vi "Poll_Data_Main_v2.vi"(8 "error in":errorcluster, 11 "Resources in":T2 {"ZI ModHandle"."ModHandle" format="0x%08x"; "ZI ModHandle"."Conn" format="0x%08x"; "ZI Handle"."Handle" format="0x%08x"; "ZI Handle"."Conn" format="0x%08x"}) -> (0 "error out":errorcluster, 1 "ZI Data 3":T1, 2 "ZI Data 0":T1, 3 "Resources out":T2 {"ZI ModHandle"."ModHandle" format="0x%08x"; "ZI ModHandle"."Conn" format="0x%08x"; "ZI Handle"."Handle" format="0x%08x"; "ZI Handle"."Conn" format="0x%08x"})   [LabVIEW 2021]
uses:
  Resources_v2.ctl
  <instrlib>/Zurich Instruments LabOne/Public/ziTypeHandle.ctl
  <instrlib>/Zurich Instruments LabOne/Public/Modules/ziTypeModHandle.ctl
  ZI_Data_v2.ctl
  <instrlib>/Zurich Instruments LabOne/Public/Modules/ziModGetDoubleData.vi
  <instrlib>/Zurich Instruments LabOne/Public/Utility/ziTicksToS_vector.vi
  <instrlib>/Zurich Instruments LabOne/Zurich Instruments LabOne.lvlib
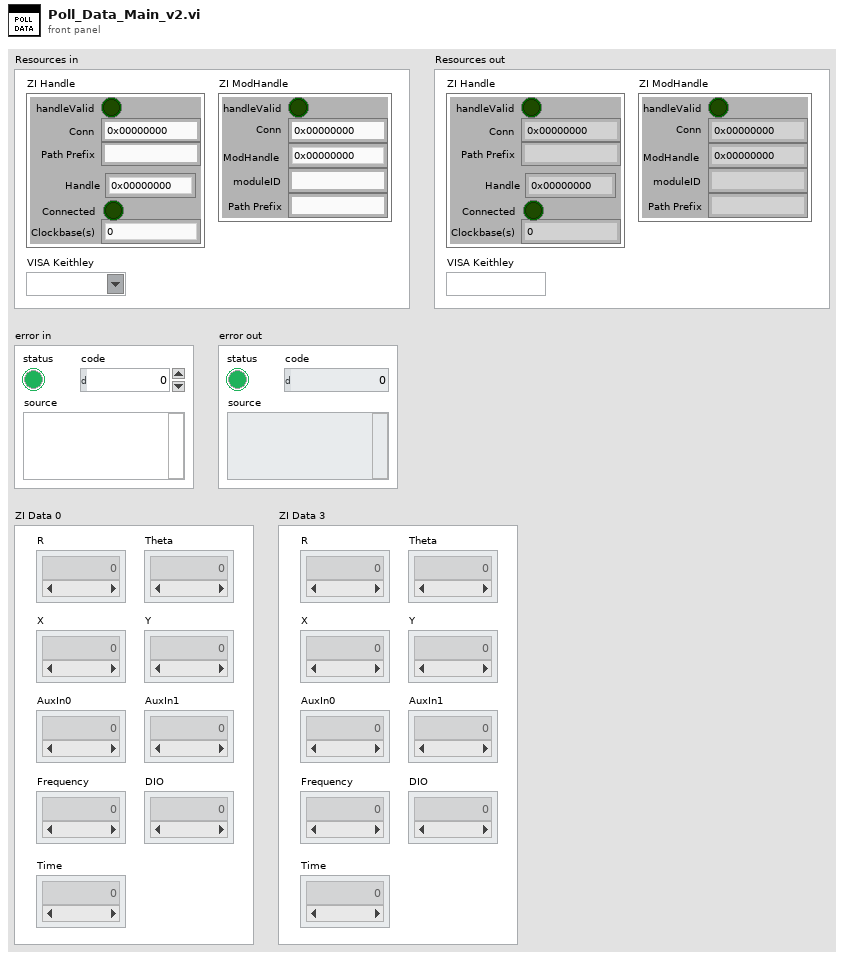
[diagram p1: front panel]
types:
  T1 = typedef "ZI_Data_v2.ctl" = cluster{"R":dbl[], "Theta":dbl[], "X":dbl[], "Y":dbl[], "AuxIn0":dbl[], "AuxIn1":dbl[], "Frequency":dbl[], "DIO":dbl[], "Time":dbl[]}
  T2 = typedef "Resources_v2.ctl" = cluster{"ZI Handle":T3, "ZI ModHandle":T4, "VISA Keithley":refnum<visa-resource-name>}
  T3 = typedef "Zurich Instruments LabOne.lvlib/ziTypeHandle.ctl" = cluster{"handleValid":bool, "Conn":u64, "Path Prefix":string, "Handle":u64, "Clockbase(s)":dbl, "Connected":bool}
  T4 = typedef "Zurich Instruments LabOne.lvlib/ziTypeModHandle.ctl" = cluster{"handleValid":bool, "Conn":u64, "ModHandle":u64, "moduleID":string, "Path Prefix":string}
  T5 = typedef "Zurich Instruments LabOne.lvlib/ziTypeModResults.ctl" = cluster{"PathArray":string[], "ValueType":T6, "NoOfResults":u64, "ziGenericHeader":T7[]}
  T6 = typedef "Zurich Instruments LabOne.lvlib/ziTypePollType.ctl" = enum16{"NONE", "DOUBLE_DATA", "INTEGER_DATA", "DEMOD_SAMPLE", "SCOPE_WAVE_HF2", "AUXIN_SAMPLE", "DIO_SAMPLE", "BYTE_ARRAY", "PWA_WAVE", "9", "10", "11", "12", "13", "14", "15", "TREE_CHANGE_DEPRI", "17", "ERROR", "19", "20", "21", "22", "23", "24", "25", "26", "27", "28", "29", "30", "31", "DOUBLE_DATA_TS", "INTEGER_DATA_TS", "34", "SCOPE_WAVE", "SCOPE_WAVE_EX", "37", "BYTE_ARRAY_TS", "39", "40", "41", "42", "43", "44", "45", "CNT_DATA", "47", "TREE_CHANGE", "49", "50", "51", "52", "53", "54", "55", "56", "57", "58", "59", "60", "61", "62", "63", "SWEEPER_DATA", "SPECTRUM_DATA", "ADVISOR_DATA", "VECTOR_DATA", "IMP_DATA"}
  T7 = typedef "Zurich Instruments LabOne.lvlib/ziTypeModGenericHeader.ctl" = cluster{"HeaderType":enum8{"HEADER_TYPE_NONE", "HEADER_TYPE_SWTRIGGER", "HEADER_TYPE_SWEEPER"}, "SampleFormat":u8, "SystemTime":timestamp, "CreatedTimeStamp":u64, "ChangedTimeStamp":u64, "Flags":u32, "ChunkSizeBytes":u64, "Name":string, "Status":u32, "GroupIndex":u32, "Color":u32, "ActiveRow":u32, "TriggerNumber":u64, "GridRows":u32, "GridCols":u32, "GridMode":u32, "GridOperation":u32, "GridDirection":u32, "GridRepetitions":u32, "GridColDelta":dbl, "GridColOffset":dbl, "GridRowDelta":dbl, "GridRowOffset":dbl, "Bandwidth":dbl, "Center":dbl, "Nenbw":dbl}
  T8 = typedef "Zurich Instruments LabOne.lvlib/ziTypeDoubleDataTS.ctl" = cluster{"Timestamp (ticks)":u64[], "Value":dbl[]}
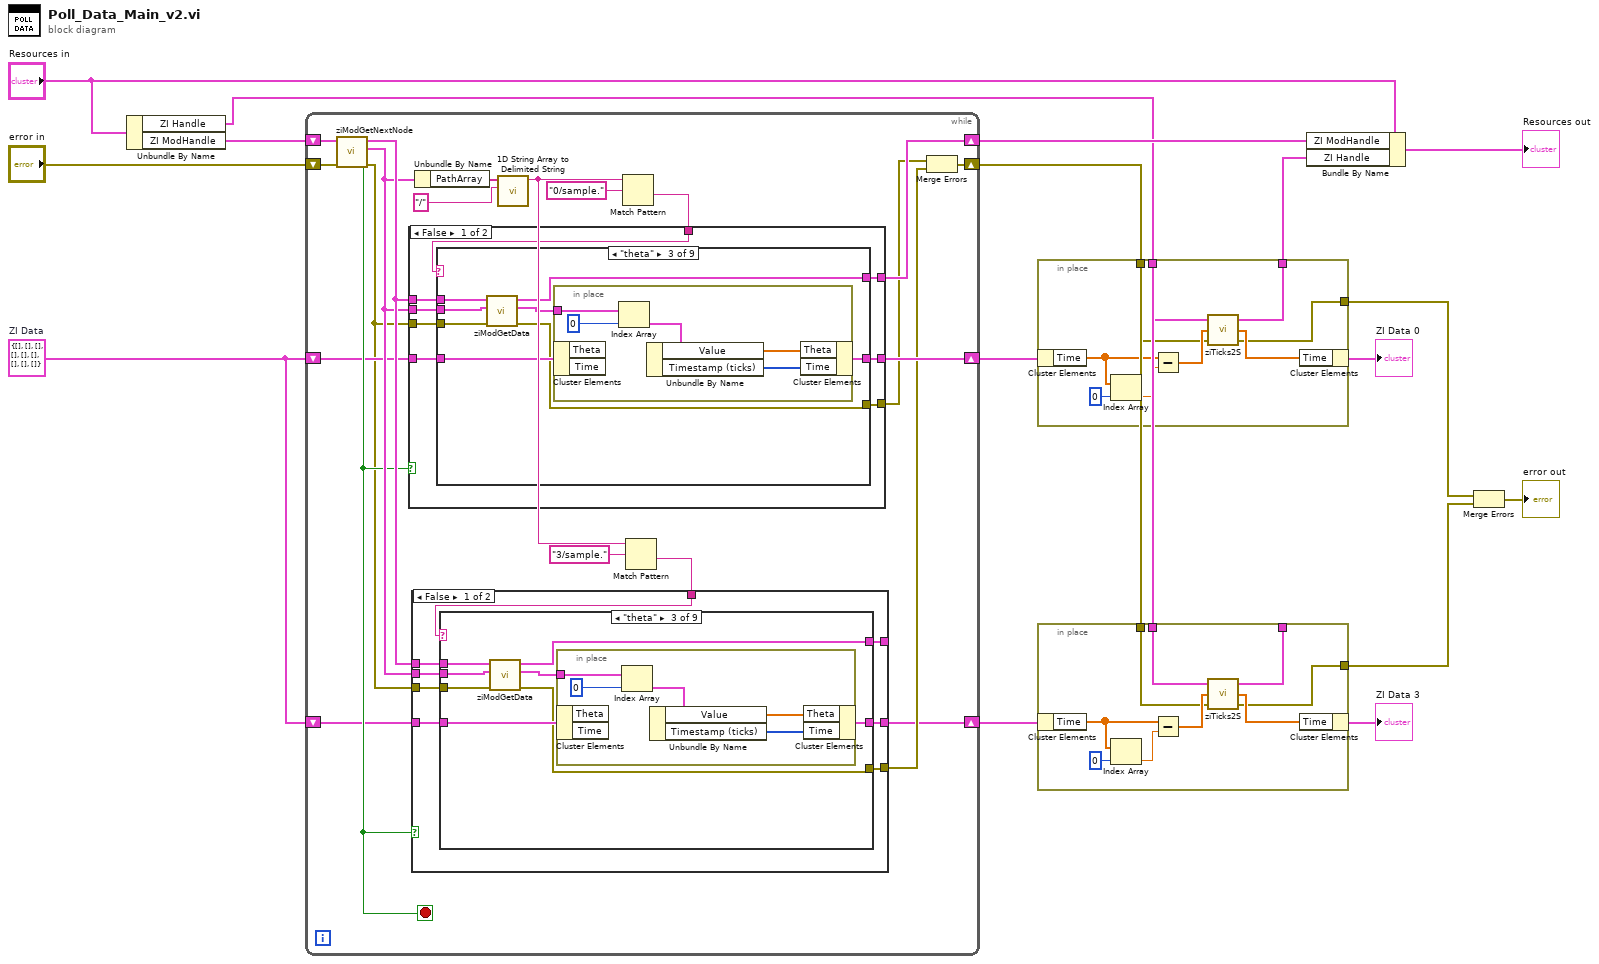
[diagram p0: block diagram]
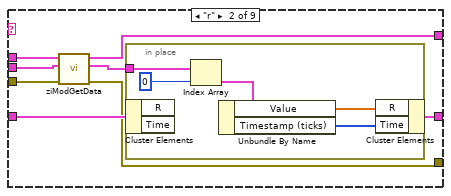
[diagram p3: hidden frame]
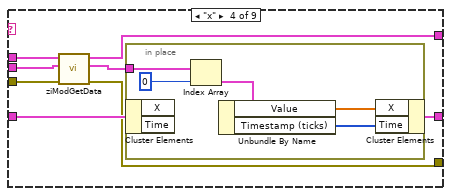
[diagram p4: hidden frame]
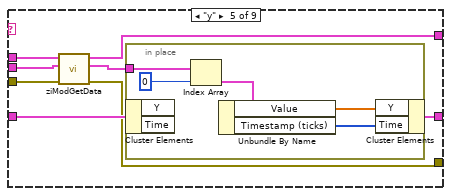
[diagram p5: hidden frame]
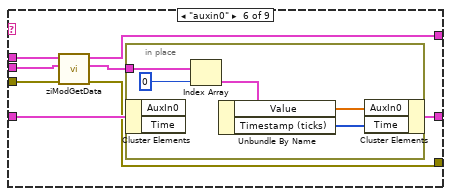
[diagram p6: hidden frame]
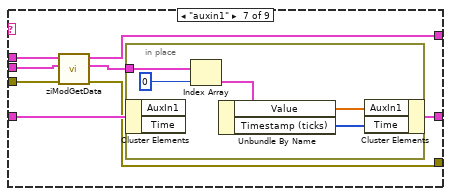
[diagram p7: hidden frame]
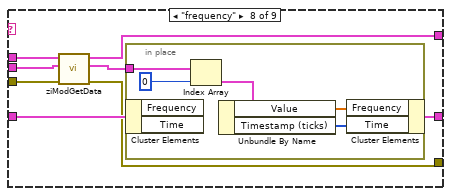
[diagram p8: hidden frame]
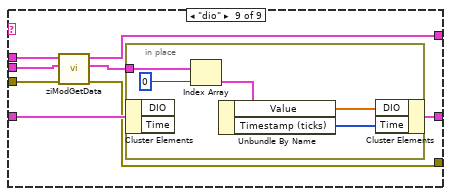
[diagram p9: hidden frame]
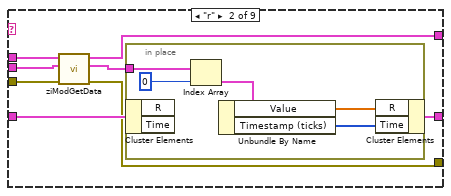
[diagram p12: hidden frame]
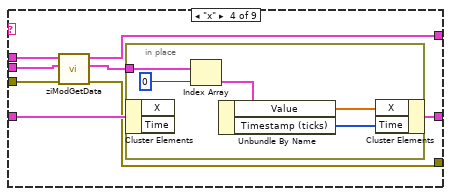
[diagram p13: hidden frame]
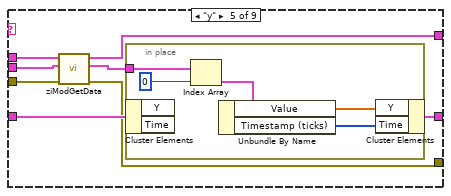
[diagram p14: hidden frame]
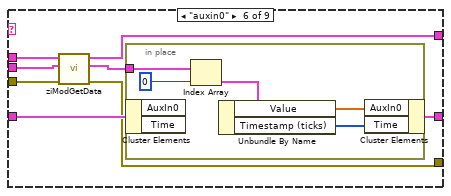
[diagram p15: hidden frame]
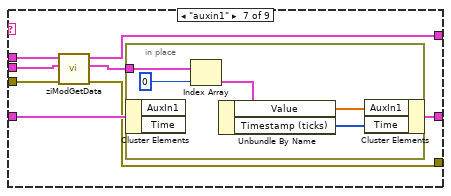
[diagram p16: hidden frame]
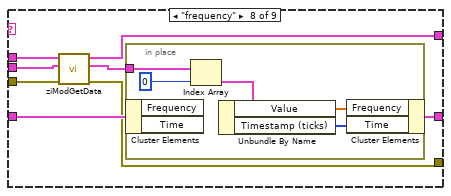
[diagram p17: hidden frame]
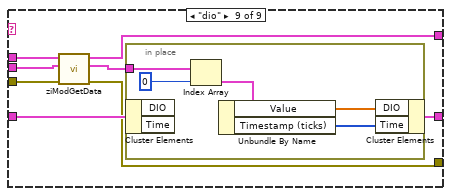
[diagram p18: hidden frame]
diagram:
  w3 = T1 {"R"=[], "Theta"=[], "X"=[], "Y"=[], "AuxIn0"=[], "AuxIn1"=[], "Frequency"=[], "DIO"=[], "Time"=[]}  # ZI Data
  n1 = Unbundle By Name("Resources in") -> ("ZI Handle"=w11:T3, "ZI ModHandle"=w13:T4)
  n2 = while {
    shift-right: [w31] -> w16
    shift-left: w13 -> [w37]
    shift-right: [w19] -> w6
    shift-left: "error in" -> [w36]
    shift-right: [w32] -> w15
    shift-left: w3 -> [w23]
    shift-right: [w17] -> w7
    shift-left: w3 -> [w18]
    stop <- w24 stop-if-true
    n3 = call <instrlib>:"ziModGetNextNode.vi"("Error In"=w36, "ModHandle In"=w37) -> ("Error Out"=w22:errorcluster, "ModResults"=w25:T5, "ModHandle Out"=w26:T4, "NoData"=w24:bool)  [unwired: 6 in]
    n4 = Unbundle By Name(w25) -> ("PathArray"=w33:string[])
    n5 = call <vilib>:"1D String Array to Delimited String.vi"("delimiter"="/", "string array"=w33) -> ("delimited string"=w27:string)  [unwired: 9 in]
    n6 = Match Pattern(string=w27, regular expression="0/sample.") -> (after substring=w30:string)  [unwired: 1 in, 3 out]
    n7 = case shown="False" w24 {
      tunnel: w30 -> [w163 _]
      tunnel: w22 -> [w161 w272]
      tunnel: w26 -> [w162 w271]
      tunnel: w25 -> [w160 _]
      tunnel: w23 -> [w159 w273]
      tunnel: [w158 w273] -> w32
      tunnel: [w157 w271] -> w31
      tunnel: [w156 w272] -> w21
      frame False {
        n8 = case shown="\"theta\"" w163 {
          tunnel: w162 -> [w166 w174 w187 w200 w213 w226 w239 w252 w265]
          tunnel: w161 -> [w164 w173 w186 w199 w212 w225 w238 w251 w264]
          tunnel: w160 -> [_ w172 w185 w198 w211 w224 w237 w250 w263]
          tunnel: w159 -> [w165 w171 w184 w197 w210 w223 w236 w249 w262]
          tunnel: [w165 w169 w182 w195 w208 w221 w234 w247 w260] -> w158
          tunnel: [w166 w168 w181 w194 w207 w220 w233 w246 w259] -> w157
          tunnel: [w164 w167 w180 w193 w206 w219 w232 w245 w258] -> w156
          frame "", Default {
          }
          frame "r" {
            n9 = call-poly <instrlib>:"ziModGetData.vi"("Error In"=w173, "ModResults"=w172, "ModHandle In"=w174) -> ("Error Out"=w167:errorcluster, "DoubleSample"=w170:T8[], "ModHandle Out"=w168:T4)  [unwired: 4 in, 2 out]
            n10 = in-place {
              in-place-border: w170 -> [w179]
              n11 = in-place-cluster #1(w171) -> ()  [unwired: 2 out]
              n12 = Index Array(array=w179, index=0) -> (element=w177:T8)
              n13 = Unbundle By Name(w177) -> ("Value"=w176:dbl[], "Timestamp (ticks)"=w175:u64[])
              n14 = in-place-cluster #1("R"=w176, "Time"=w175) -> (w169:T1)
            }
          }
          frame "theta" {
            n15 = call-poly <instrlib>:"ziModGetData.vi"("Error In"=w186, "ModResults"=w185, "ModHandle In"=w187) -> ("Error Out"=w180:errorcluster, "DoubleSample"=w183:T8[], "ModHandle Out"=w181:T4)  [unwired: 4 in, 2 out]
            n16 = in-place {
              in-place-border: w183 -> [w192]
              n17 = in-place-cluster #2(w184) -> ()  [unwired: 2 out]
              n18 = Index Array(array=w192, index=0) -> (element=w190:T8)
              n19 = Unbundle By Name(w190) -> ("Value"=w189:dbl[], "Timestamp (ticks)"=w188:u64[])
              n20 = in-place-cluster #2("Theta"=w189, "Time"=w188) -> (w182:T1)
            }
          }
          frame "x" {
            n21 = call-poly <instrlib>:"ziModGetData.vi"("Error In"=w199, "ModResults"=w198, "ModHandle In"=w200) -> ("Error Out"=w193:errorcluster, "DoubleSample"=w196:T8[], "ModHandle Out"=w194:T4)  [unwired: 4 in, 2 out]
            n22 = in-place {
              in-place-border: w196 -> [w205]
              n23 = in-place-cluster #3(w197) -> ()  [unwired: 2 out]
              n24 = Index Array(array=w205, index=0) -> (element=w203:T8)
              n25 = Unbundle By Name(w203) -> ("Value"=w202:dbl[], "Timestamp (ticks)"=w201:u64[])
              n26 = in-place-cluster #3("X"=w202, "Time"=w201) -> (w195:T1)
            }
          }
          frame "y" {
            n27 = call-poly <instrlib>:"ziModGetData.vi"("Error In"=w212, "ModResults"=w211, "ModHandle In"=w213) -> ("Error Out"=w206:errorcluster, "DoubleSample"=w209:T8[], "ModHandle Out"=w207:T4)  [unwired: 4 in, 2 out]
            n28 = in-place {
              in-place-border: w209 -> [w218]
              n29 = in-place-cluster #4(w210) -> ()  [unwired: 2 out]
              n30 = Index Array(array=w218, index=0) -> (element=w216:T8)
              n31 = Unbundle By Name(w216) -> ("Value"=w215:dbl[], "Timestamp (ticks)"=w214:u64[])
              n32 = in-place-cluster #4("Y"=w215, "Time"=w214) -> (w208:T1)
            }
          }
          frame "auxin0" {
            n33 = call-poly <instrlib>:"ziModGetData.vi"("Error In"=w225, "ModResults"=w224, "ModHandle In"=w226) -> ("Error Out"=w219:errorcluster, "DoubleSample"=w222:T8[], "ModHandle Out"=w220:T4)  [unwired: 4 in, 2 out]
            n34 = in-place {
              in-place-border: w222 -> [w231]
              n35 = in-place-cluster #5(w223) -> ()  [unwired: 2 out]
              n36 = Index Array(array=w231, index=0) -> (element=w229:T8)
              n37 = Unbundle By Name(w229) -> ("Value"=w228:dbl[], "Timestamp (ticks)"=w227:u64[])
              n38 = in-place-cluster #5("AuxIn0"=w228, "Time"=w227) -> (w221:T1)
            }
          }
          frame "auxin1" {
            n39 = call-poly <instrlib>:"ziModGetData.vi"("Error In"=w238, "ModResults"=w237, "ModHandle In"=w239) -> ("Error Out"=w232:errorcluster, "DoubleSample"=w235:T8[], "ModHandle Out"=w233:T4)  [unwired: 4 in, 2 out]
            n40 = in-place {
              in-place-border: w235 -> [w244]
              n41 = in-place-cluster #6(w236) -> ()  [unwired: 2 out]
              n42 = Index Array(array=w244, index=0) -> (element=w242:T8)
              n43 = Unbundle By Name(w242) -> ("Value"=w241:dbl[], "Timestamp (ticks)"=w240:u64[])
              n44 = in-place-cluster #6("AuxIn1"=w241, "Time"=w240) -> (w234:T1)
            }
          }
          frame "frequency" {
            n45 = call-poly <instrlib>:"ziModGetData.vi"("Error In"=w251, "ModResults"=w250, "ModHandle In"=w252) -> ("Error Out"=w245:errorcluster, "DoubleSample"=w248:T8[], "ModHandle Out"=w246:T4)  [unwired: 4 in, 2 out]
            n46 = in-place {
              in-place-border: w248 -> [w257]
              n47 = in-place-cluster #7(w249) -> ()  [unwired: 2 out]
              n48 = Index Array(array=w257, index=0) -> (element=w255:T8)
              n49 = Unbundle By Name(w255) -> ("Value"=w254:dbl[], "Timestamp (ticks)"=w253:u64[])
              n50 = in-place-cluster #7("Frequency"=w254, "Time"=w253) -> (w247:T1)
            }
          }
          frame "dio" {
            n51 = call-poly <instrlib>:"ziModGetData.vi"("Error In"=w264, "ModResults"=w263, "ModHandle In"=w265) -> ("Error Out"=w258:errorcluster, "DoubleSample"=w261:T8[], "ModHandle Out"=w259:T4)  [unwired: 4 in, 2 out]
            n52 = in-place {
              in-place-border: w261 -> [w270]
              n53 = in-place-cluster #8(w262) -> ()  [unwired: 2 out]
              n54 = Index Array(array=w270, index=0) -> (element=w268:T8)
              n55 = Unbundle By Name(w268) -> ("Value"=w267:dbl[], "Timestamp (ticks)"=w266:u64[])
              n56 = in-place-cluster #8("DIO"=w267, "Time"=w266) -> (w260:T1)
            }
          }
        }
      }
      frame True {
      }
    }
    n57 = Match Pattern(string=w27, regular expression="3/sample.") -> (after substring=w29:string)  [unwired: 1 in, 3 out]
    n58 = case shown="False" w24 {
      tunnel: w29 -> [w45 _]
      tunnel: w22 -> [w43 w154]
      tunnel: w26 -> [w44 w153]
      tunnel: w25 -> [w42 _]
      tunnel: w18 -> [w41 w155]
      tunnel: [w40 w155] -> w17
      tunnel: [w39 w153] -> _
      tunnel: [w38 w154] -> w20
      frame False {
        n59 = case shown="\"theta\"" w45 {
          tunnel: w44 -> [w48 w56 w69 w82 w95 w108 w121 w134 w147]
          tunnel: w43 -> [w46 w55 w68 w81 w94 w107 w120 w133 w146]
          tunnel: w42 -> [_ w54 w67 w80 w93 w106 w119 w132 w145]
          tunnel: w41 -> [w47 w53 w66 w79 w92 w105 w118 w131 w144]
          tunnel: [w47 w51 w64 w77 w90 w103 w116 w129 w142] -> w40
          tunnel: [w48 w50 w63 w76 w89 w102 w115 w128 w141] -> w39
          tunnel: [w46 w49 w62 w75 w88 w101 w114 w127 w140] -> w38
          frame "", Default {
          }
          frame "r" {
            n60 = call-poly <instrlib>:"ziModGetData.vi"("Error In"=w55, "ModResults"=w54, "ModHandle In"=w56) -> ("Error Out"=w49:errorcluster, "DoubleSample"=w52:T8[], "ModHandle Out"=w50:T4)  [unwired: 4 in, 2 out]
            n61 = in-place {
              in-place-border: w52 -> [w61]
              n62 = in-place-cluster #9(w53) -> ()  [unwired: 2 out]
              n63 = Index Array(array=w61, index=0) -> (element=w59:T8)
              n64 = Unbundle By Name(w59) -> ("Value"=w58:dbl[], "Timestamp (ticks)"=w57:u64[])
              n65 = in-place-cluster #9("R"=w58, "Time"=w57) -> (w51:T1)
            }
          }
          frame "theta" {
            n66 = call-poly <instrlib>:"ziModGetData.vi"("Error In"=w68, "ModResults"=w67, "ModHandle In"=w69) -> ("Error Out"=w62:errorcluster, "DoubleSample"=w65:T8[], "ModHandle Out"=w63:T4)  [unwired: 4 in, 2 out]
            n67 = in-place {
              in-place-border: w65 -> [w74]
              n68 = in-place-cluster #10(w66) -> ()  [unwired: 2 out]
              n69 = Index Array(array=w74, index=0) -> (element=w72:T8)
              n70 = Unbundle By Name(w72) -> ("Value"=w71:dbl[], "Timestamp (ticks)"=w70:u64[])
              n71 = in-place-cluster #10("Theta"=w71, "Time"=w70) -> (w64:T1)
            }
          }
          frame "x" {
            n72 = call-poly <instrlib>:"ziModGetData.vi"("Error In"=w81, "ModResults"=w80, "ModHandle In"=w82) -> ("Error Out"=w75:errorcluster, "DoubleSample"=w78:T8[], "ModHandle Out"=w76:T4)  [unwired: 4 in, 2 out]
            n73 = in-place {
              in-place-border: w78 -> [w87]
              n74 = in-place-cluster #11(w79) -> ()  [unwired: 2 out]
              n75 = Index Array(array=w87, index=0) -> (element=w85:T8)
              n76 = Unbundle By Name(w85) -> ("Value"=w84:dbl[], "Timestamp (ticks)"=w83:u64[])
              n77 = in-place-cluster #11("X"=w84, "Time"=w83) -> (w77:T1)
            }
          }
          frame "y" {
            n78 = call-poly <instrlib>:"ziModGetData.vi"("Error In"=w94, "ModResults"=w93, "ModHandle In"=w95) -> ("Error Out"=w88:errorcluster, "DoubleSample"=w91:T8[], "ModHandle Out"=w89:T4)  [unwired: 4 in, 2 out]
            n79 = in-place {
              in-place-border: w91 -> [w100]
              n80 = in-place-cluster #12(w92) -> ()  [unwired: 2 out]
              n81 = Index Array(array=w100, index=0) -> (element=w98:T8)
              n82 = Unbundle By Name(w98) -> ("Value"=w97:dbl[], "Timestamp (ticks)"=w96:u64[])
              n83 = in-place-cluster #12("Y"=w97, "Time"=w96) -> (w90:T1)
            }
          }
          frame "auxin0" {
            n84 = call-poly <instrlib>:"ziModGetData.vi"("Error In"=w107, "ModResults"=w106, "ModHandle In"=w108) -> ("Error Out"=w101:errorcluster, "DoubleSample"=w104:T8[], "ModHandle Out"=w102:T4)  [unwired: 4 in, 2 out]
            n85 = in-place {
              in-place-border: w104 -> [w113]
              n86 = in-place-cluster #13(w105) -> ()  [unwired: 2 out]
              n87 = Index Array(array=w113, index=0) -> (element=w111:T8)
              n88 = Unbundle By Name(w111) -> ("Value"=w110:dbl[], "Timestamp (ticks)"=w109:u64[])
              n89 = in-place-cluster #13("AuxIn0"=w110, "Time"=w109) -> (w103:T1)
            }
          }
          frame "auxin1" {
            n90 = call-poly <instrlib>:"ziModGetData.vi"("Error In"=w120, "ModResults"=w119, "ModHandle In"=w121) -> ("Error Out"=w114:errorcluster, "DoubleSample"=w117:T8[], "ModHandle Out"=w115:T4)  [unwired: 4 in, 2 out]
            n91 = in-place {
              in-place-border: w117 -> [w126]
              n92 = in-place-cluster #14(w118) -> ()  [unwired: 2 out]
              n93 = Index Array(array=w126, index=0) -> (element=w124:T8)
              n94 = Unbundle By Name(w124) -> ("Value"=w123:dbl[], "Timestamp (ticks)"=w122:u64[])
              n95 = in-place-cluster #14("AuxIn1"=w123, "Time"=w122) -> (w116:T1)
            }
          }
          frame "frequency" {
            n96 = call-poly <instrlib>:"ziModGetData.vi"("Error In"=w133, "ModResults"=w132, "ModHandle In"=w134) -> ("Error Out"=w127:errorcluster, "DoubleSample"=w130:T8[], "ModHandle Out"=w128:T4)  [unwired: 4 in, 2 out]
            n97 = in-place {
              in-place-border: w130 -> [w139]
              n98 = in-place-cluster #15(w131) -> ()  [unwired: 2 out]
              n99 = Index Array(array=w139, index=0) -> (element=w137:T8)
              n100 = Unbundle By Name(w137) -> ("Value"=w136:dbl[], "Timestamp (ticks)"=w135:u64[])
              n101 = in-place-cluster #15("Frequency"=w136, "Time"=w135) -> (w129:T1)
            }
          }
          frame "dio" {
            n102 = call-poly <instrlib>:"ziModGetData.vi"("Error In"=w146, "ModResults"=w145, "ModHandle In"=w147) -> ("Error Out"=w140:errorcluster, "DoubleSample"=w143:T8[], "ModHandle Out"=w141:T4)  [unwired: 4 in, 2 out]
            n103 = in-place {
              in-place-border: w143 -> [w152]
              n104 = in-place-cluster #16(w144) -> ()  [unwired: 2 out]
              n105 = Index Array(array=w152, index=0) -> (element=w150:T8)
              n106 = Unbundle By Name(w150) -> ("Value"=w149:dbl[], "Timestamp (ticks)"=w148:u64[])
              n107 = in-place-cluster #16("DIO"=w149, "Time"=w148) -> (w142:T1)
            }
          }
        }
      }
      frame True {
      }
    }
    n108 = Merge Errors(w21, w20) -> (w19:errorcluster)
  }
  n109 = in-place {
    in-place-border: w11 -> [w279]
    in-place-border: [w276] -> w14
    in-place-border: w6 -> [w275]
    in-place-border: [w274] -> w9
    n110 = in-place-cluster #17(w15) -> ("Time"=w280:dbl[])
    n111 = Index Array(array=w280, index=0) -> (element=w281:dbl)
    n112 = Subtract(x=w280, y=w281) -> (x-y=w278:dbl[])
    n113 = call-poly <instrlib>:"ziTicks2S.vi"("Error In"=w275, "Timestamp (ticks)"=w278, "Handle In"=w279) -> ("Error Out"=w274:errorcluster, "Timestamp(s)"=w277:dbl[], "Handle Out"=w276:T3)
    n114 = in-place-cluster #17("Time"=w277) -> (→"ZI Data 0":T1)
  }
  n115 = in-place {
    in-place-border: w11 -> [w288]
    in-place-border: [w285] -> _
    in-place-border: w6 -> [w284]
    in-place-border: [w283] -> w8
    n116 = in-place-cluster #18(w7) -> ("Time"=w289:dbl[])
    n117 = Index Array(array=w289, index=0) -> (element=w290:dbl)
    n118 = Subtract(x=w289, y=w290) -> (x-y=w287:dbl[])
    n119 = call-poly <instrlib>:"ziTicks2S.vi"("Error In"=w284, "Timestamp (ticks)"=w287, "Handle In"=w288) -> ("Error Out"=w283:errorcluster, "Timestamp(s)"=w286:dbl[], "Handle Out"=w285:T3)
    n120 = in-place-cluster #18("Time"=w286) -> (→"ZI Data 3":T1)
  }
  n121 = Bundle By Name(cluster="Resources in", "ZI ModHandle"=w16, "ZI Handle"=w14) -> (→"Resources out":T2)
  n122 = Merge Errors(w9, w8) -> (→"error out":errorcluster)
